vi "Create_DO_Module.vi"(8 "error in (no error)":errorcluster) -> (0 "error out":errorcluster)   [LabVIEW 2019, in "USB-87Pn.lvlib" / "USB-87Pn.lvclass"]
uses:
  USB-87Pn.lvclass
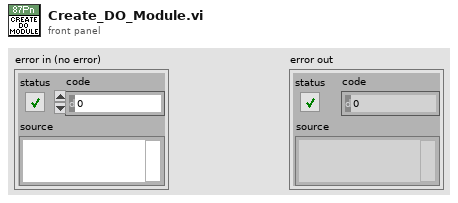
[diagram p1: front panel]
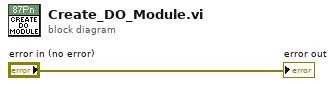
[diagram p0: block diagram]
diagram:
  "error out" <- "error in (no error)"
